vi "main.vi"() -> ()   [LabVIEW 2015]
uses:
  <vilib>/Instr/_visa.llb/VISA Configure Serial Port (Instr).vi
panel:
  out "波形图表":cluster{sgl, sgl}(graph)
  out "send flag":bool
  in  "baud rate":u64(ring) items=["9600"=9600, "14400"=14400, "115200"=115200]
  out "read buffer":string
  out "serial_state":bool
  in  "serial":refnum<visa-resource-name> caption="serial_select"
  in  "serial_open":bool
  in  "exit":bool
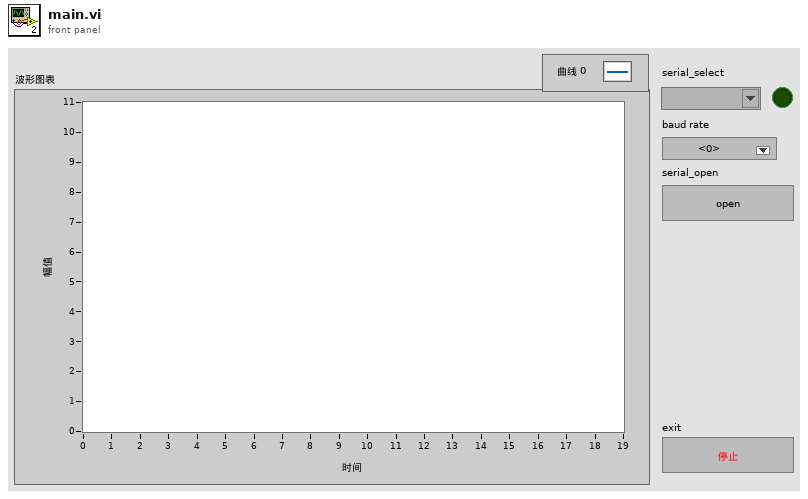
[diagram p1: front panel]
types:
  T1 = typedef "状态机.ctl" = enum16{"Init", "Wait", "Send", "GetData", "Deal", "Exit"}
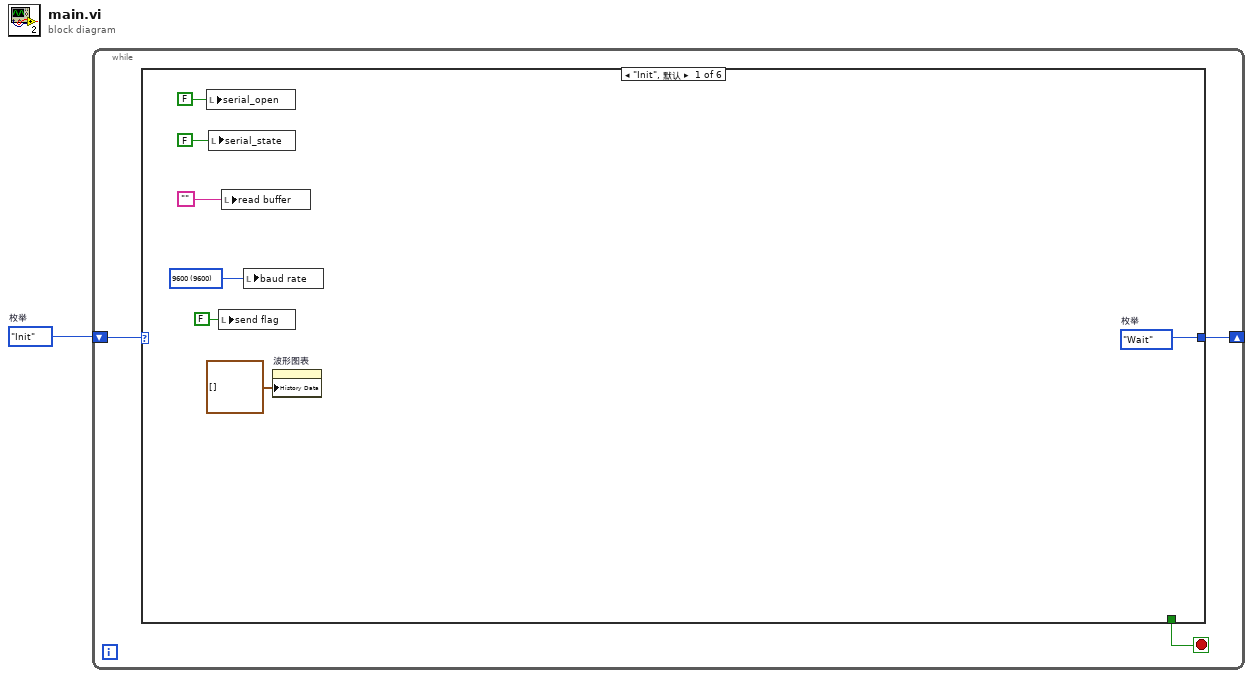
[diagram p0: block diagram]
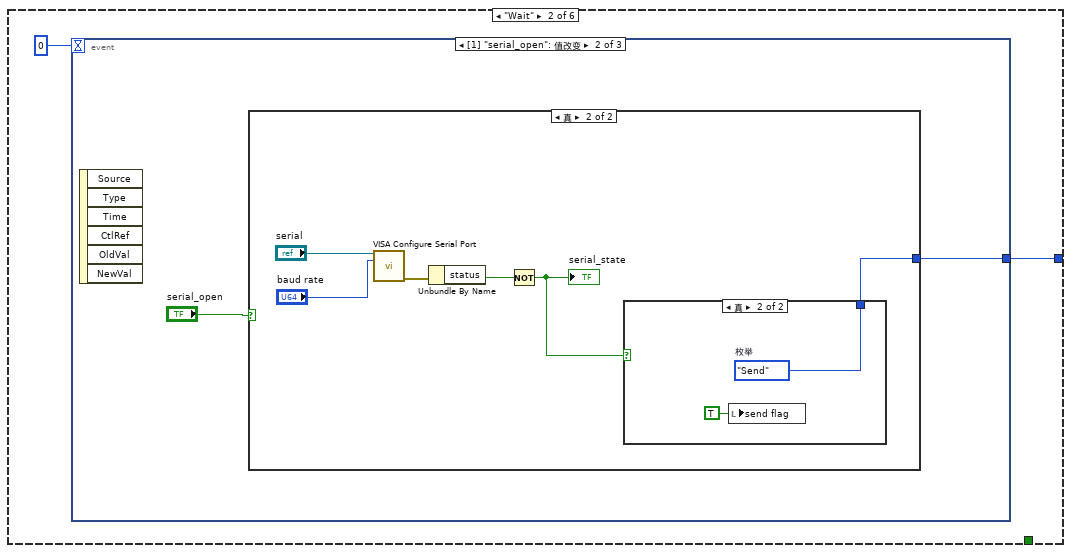
[diagram p2: hidden frame]
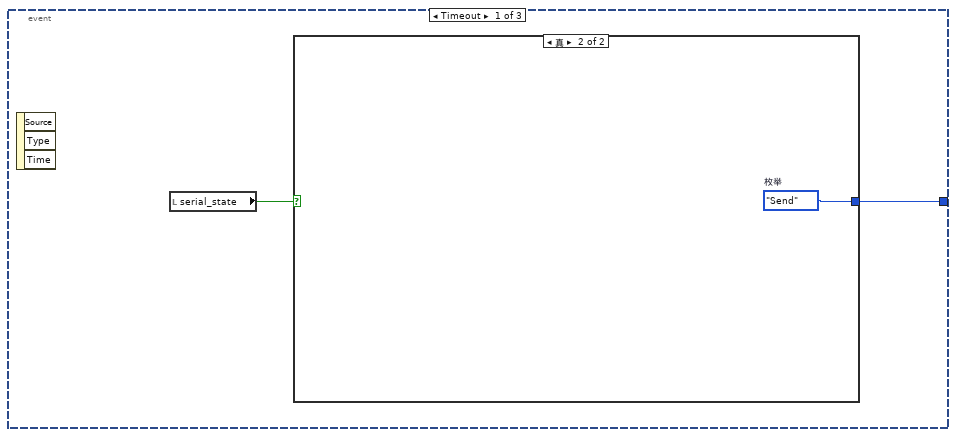
[diagram p3: hidden frame]
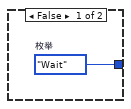
[diagram p4: hidden frame]
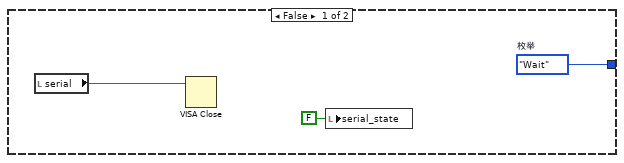
[diagram p5: hidden frame]
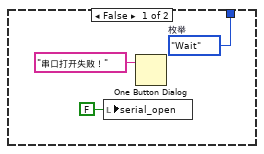
[diagram p6: hidden frame]
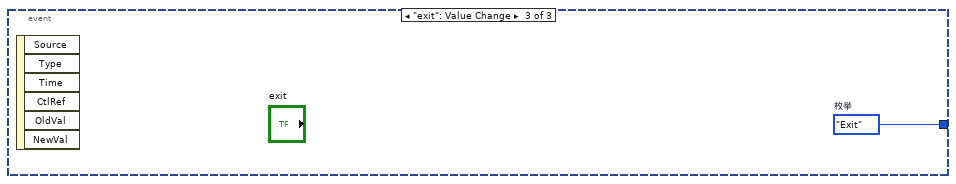
[diagram p7: hidden frame]
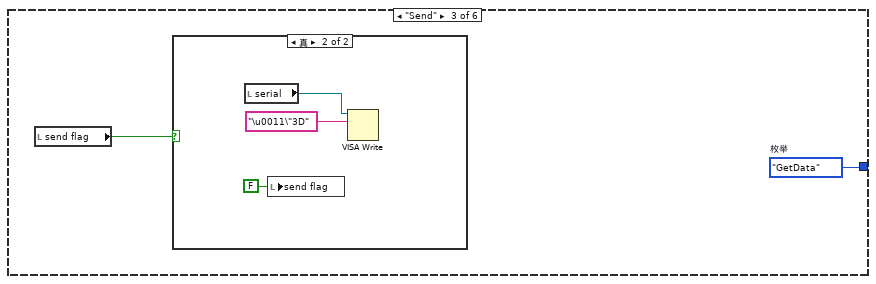
[diagram p8: hidden frame]
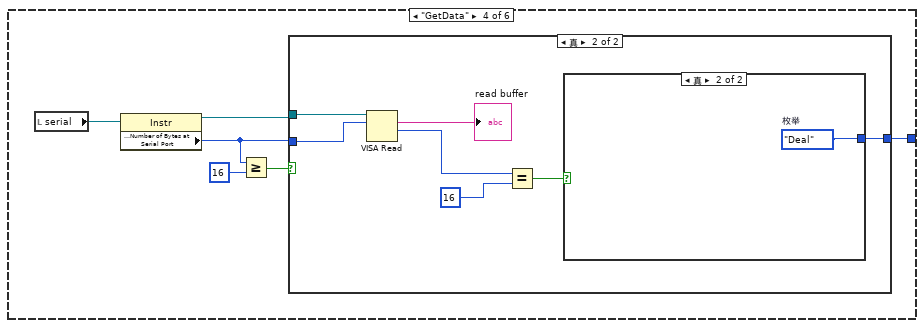
[diagram p10: hidden frame]
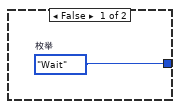
[diagram p11: hidden frame]
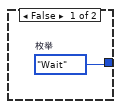
[diagram p12: hidden frame]
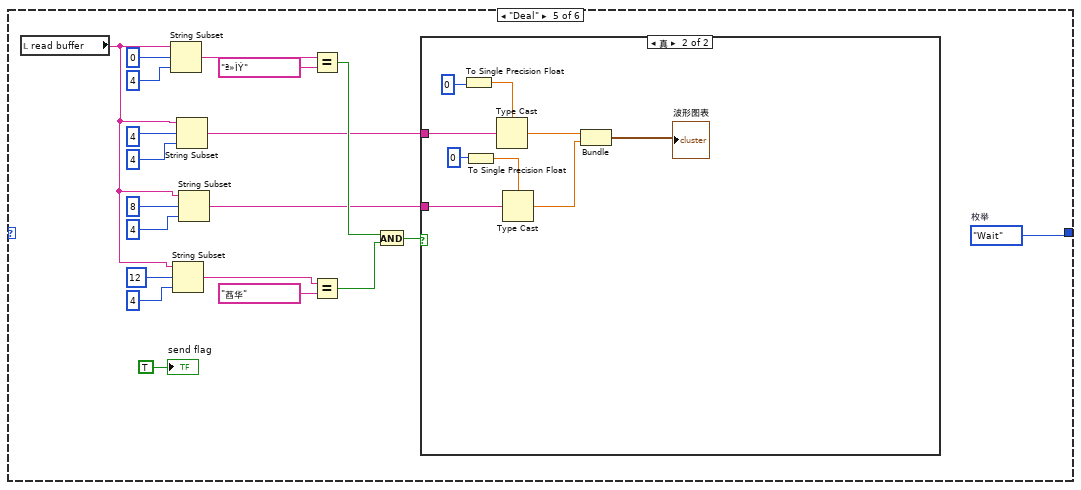
[diagram p13: hidden frame]
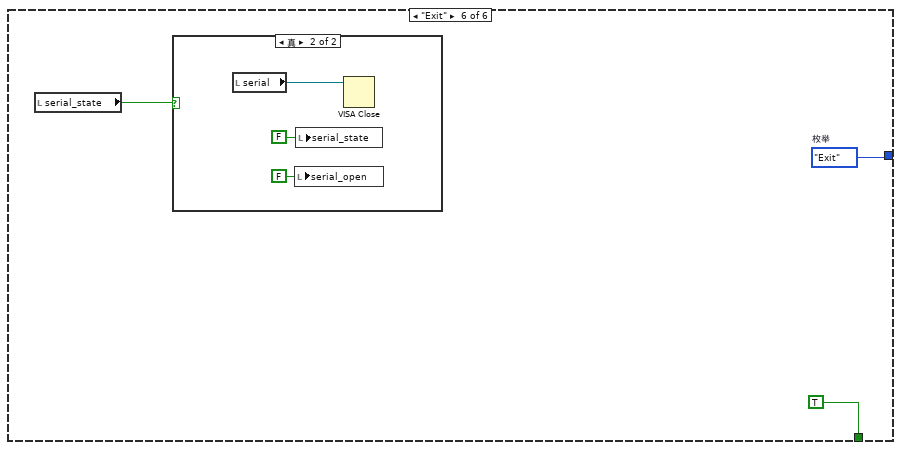
[diagram p15: hidden frame]
diagram:
  w1 = 状态机."Init"  # 枚举
  n1 = while {
    shift-right: [w3] -> _
    shift-left: w1 -> [w4]
    stop <- w2 stop-if-true
    n2 = case shown="\"Init\", 默认" w4 {
      tunnel: [w9 w12 w36 w43 w75 w87] -> w3
      tunnel: [_ _ _ _ _ TRUE] -> w2
      frame "Init", Default {
        w7 = u64 9600 items=["9600"=9600, "115200"=115200] ("baud rate")
        w9 = 状态机."Wait"  # 枚举
        n3 = local write "serial_open"(FALSE ("serial_open")) -> ()
        n4 = local write "serial_state"(FALSE ("serial_state")) -> ()
        n5 = local write "send flag"(FALSE ("send flag")) -> ()
        n6 = local write "read buffer"("") -> ()
        n7 = local write "baud rate"(w7) -> ()
        n8 = property on="波形图表" class="WFChart (严格)"("History Data"=cluster{u32, u32}[] [] ("历史数据")) -> ()  [unwired: 2 in, 2 out]
      }
      frame "Wait" {
        n9 = event shown="[1] \"serial_open\": 值改变" {
          selector: _ -> [_ _ _]
          dyn-events: _ -> [_ _ _]
          timeout: 0 -> [_ _ _]
          tunnel: [w14 w18 w34] -> w12
          event Timeout {
            n10 = event-data() -> ()  [unwired: 1 in, 3 out]
            n11 = local read "serial_state"() -> (w15:bool)
            n12 = case shown="真" w15 {
              tunnel: [w16 w17] -> w14
              frame False {
                w16 = 状态机."Wait"  # 枚举
              }
              frame True {
                w17 = 状态机."Send"  # 枚举
              }
            }
          }
          event "serial_open": Value Change {
            n13 = event-data() -> ()  [unwired: 1 in, 6 out]
            n14 = case shown="真" "serial_open" {
              tunnel: [w20 w24] -> w18
              frame False {
                w20 = 状态机."Wait"  # 枚举
                n15 = local read "serial"() -> (w22:refnum<visa-resource-name>)
                n16 = VISA Close(VISA resource name=w22) -> ()  [unwired: 1 in, 1 out]
                n17 = local write "serial_state"(FALSE ("serial_state")) -> ()
              }
              frame True {
                n18 = call-poly "VISA Configure Serial Port"("VISA resource name"="serial", "baud rate (9600)"="baud rate") -> ("error out"=w27:errorcluster)  [unwired: 12 in, 1 out]
                n19 = Unbundle By Name(w27) -> ("status"=w26:bool)
                n20 = Not(x=w26) -> (.not. x?=w25:bool)
                "serial_state" <- w25
                n21 = case shown="真" w25 {
                  tunnel: [w29 w33] -> w24
                  frame False {
                    w29 = 状态机."Wait"  # 枚举
                    n22 = local write "serial_open"(FALSE ("serial_open")) -> ()
                    n23 = One Button Dialog(message="串口打开失败！" ("消息")) -> ()  [unwired: 1 in, 1 out]
                  }
                  frame True {
                    w33 = 状态机."Send"  # 枚举
                    n24 = local write "send flag"(TRUE ("send flag")) -> ()
                  }
                }
              }
            }
          }
          event "exit": Value Change {
            w34 = 状态机."Exit"  # 枚举
            n25 = event-data() -> ()  [unwired: 1 in, 6 out]
          }
        }
      }
      frame "Send" {
        w36 = 状态机."GetData"  # 枚举
        n26 = local read "send flag"() -> (w35:bool)
        n27 = case shown="真" w35 {
          frame False {
          }
          frame True {
            n28 = local read "serial"() -> (w38:refnum<visa-resource-name>)
            n29 = local write "send flag"(FALSE ("send flag")) -> ()
            n30 = VISA Write(VISA resource name=w38, write buffer="\u0011\"3D" ("写入缓冲区")) -> ()  [unwired: 1 in, 3 out]
          }
        }
      }
      frame "GetData" {
        n31 = local read "serial"() -> (w44:refnum<visa-resource-name>)
        n32 = property class="Instr"(reference=w44) -> (reference out=w45:refnum<visa-resource-name>, "Serial Settings:Number of Bytes at Serial Port"=w41:u32)  [unwired: 1 in, 1 out]
        n33 = Greater Or Equal?(x=w41, y=u32 16) -> (x >= y?=w42:bool)
        n34 = case shown="真" w42 {
          tunnel: w45 -> [_ w53]
          tunnel: w41 -> [_ w52]
          tunnel: [w46 w47] -> w43
          frame False {
            w46 = 状态机."Wait"  # 枚举
          }
          frame True {
            n35 = VISA Read(VISA resource name=w53, byte count=w52) -> (read buffer=→"read buffer":string, return count=w50:u32)  [unwired: 1 in, 2 out]
            n36 = Equal?(x=w50, y=u32 16) -> (x = y?=w48:bool)
            n37 = case shown="真" w48 {
              tunnel: [w54 w55] -> w47
              frame False {
                w54 = 状态机."Wait"  # 枚举
              }
              frame True {
                w55 = 状态机."Deal"  # 枚举
              }
            }
          }
        }
      }
      frame "Deal" {
        w75 = 状态机."Wait"  # 枚举
        n38 = local read "read buffer"() -> (w57:string)
        n39 = String Subset(string=w57, offset (0)=0 ("偏移量(0)"), length (rest)=4 ("长度（剩余）")) -> (substring=w68:string)
        n40 = String Subset(string=w57, offset (0)=12 ("偏移量(0)"), length (rest)=4 ("长度（剩余）")) -> (substring=w65:string)
        n41 = String Subset(string=w57, offset (0)=4 ("偏移量(0)"), length (rest)=4 ("长度（剩余）")) -> (substring=w61:string)
        n42 = String Subset(string=w57, offset (0)=8 ("偏移量(0)"), length (rest)=4 ("长度（剩余）")) -> (substring=w56:string)
        n43 = Equal?(x=w68, y="ª»ÌÝ") -> (x = y?=w63:bool)
        n44 = Equal?(x=w65, y="萏华") -> (x = y?=w62:bool)
        n45 = And(x=w63, y=w62) -> (x .and. y?=w64:bool)
        n46 = case shown="真" w64 {
          tunnel: w61 -> [_ w84]
          tunnel: w56 -> [_ w83]
          frame False {
          }
          frame True {
            n47 = To Single Precision Float(number=0) -> (single precision float=w78:sgl)
            n48 = To Single Precision Float(number=0) -> (single precision float=w76:sgl)
            n49 = Type Cast(type=w78, x=w84) -> (*(type *) &x=w82:sgl)
            n50 = Type Cast(type=w76, x=w83) -> (*(type *) &x=w81:sgl)
            n51 = Bundle(w82, w81) -> (→"波形图表":cluster{sgl, sgl})  [unwired: 1 in]
          }
        }
        "send flag" <- TRUE ("send flag")
      }
      frame "Exit" {
        w87 = 状态机."Exit"  # 枚举
        n52 = local read "serial_state"() -> (w85:bool)
        n53 = case shown="真" w85 {
          frame False {
          }
          frame True {
            n54 = local read "serial"() -> (w90:refnum<visa-resource-name>)
            n55 = local write "serial_open"(FALSE ("serial_state")) -> ()
            n56 = local write "serial_state"(FALSE ("serial_state")) -> ()
            n57 = VISA Close(VISA resource name=w90) -> ()  [unwired: 1 in, 1 out]
          }
        }
      }
    }
  }
